vi "Move_Arm_to_Card_Pickup3.vi"(9 "index":i32=19, 10 "error in":errorcluster, 11 "Machine In":refnum<visa-resource-name>) -> (0 "X Coordinate":dbl, 1 "Y Coordinate":dbl, 2 "error out":errorcluster, 3 "Machine Out":refnum<visa-resource-name>, 4 "Z Coordinate":dbl=5.0)   [LabVIEW 2018]
doc: "Example interface for controlling uArm Swift Pro."
panel:
  in  "Write Buffer":string="G90 G0 X1\n"
  out "read buffer":string
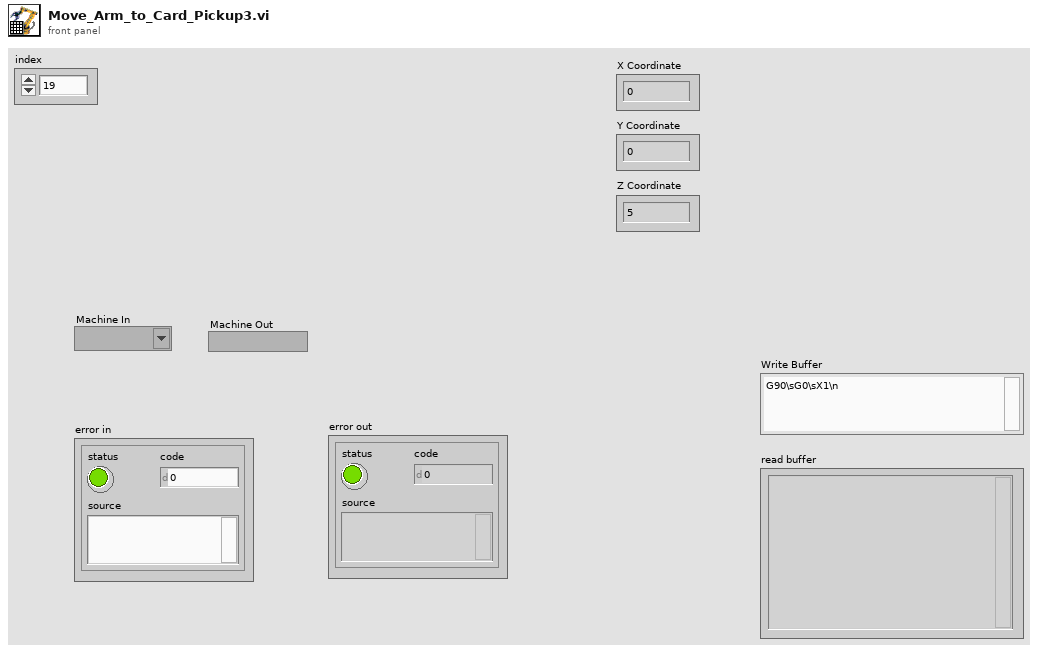
[diagram p1: front panel]
types:
  T1 = cluster{"Numeric Control":dbl, "Numeric Control":dbl}[]
  T2 = cluster{"Numeric Control":dbl, "Numeric Control":dbl}
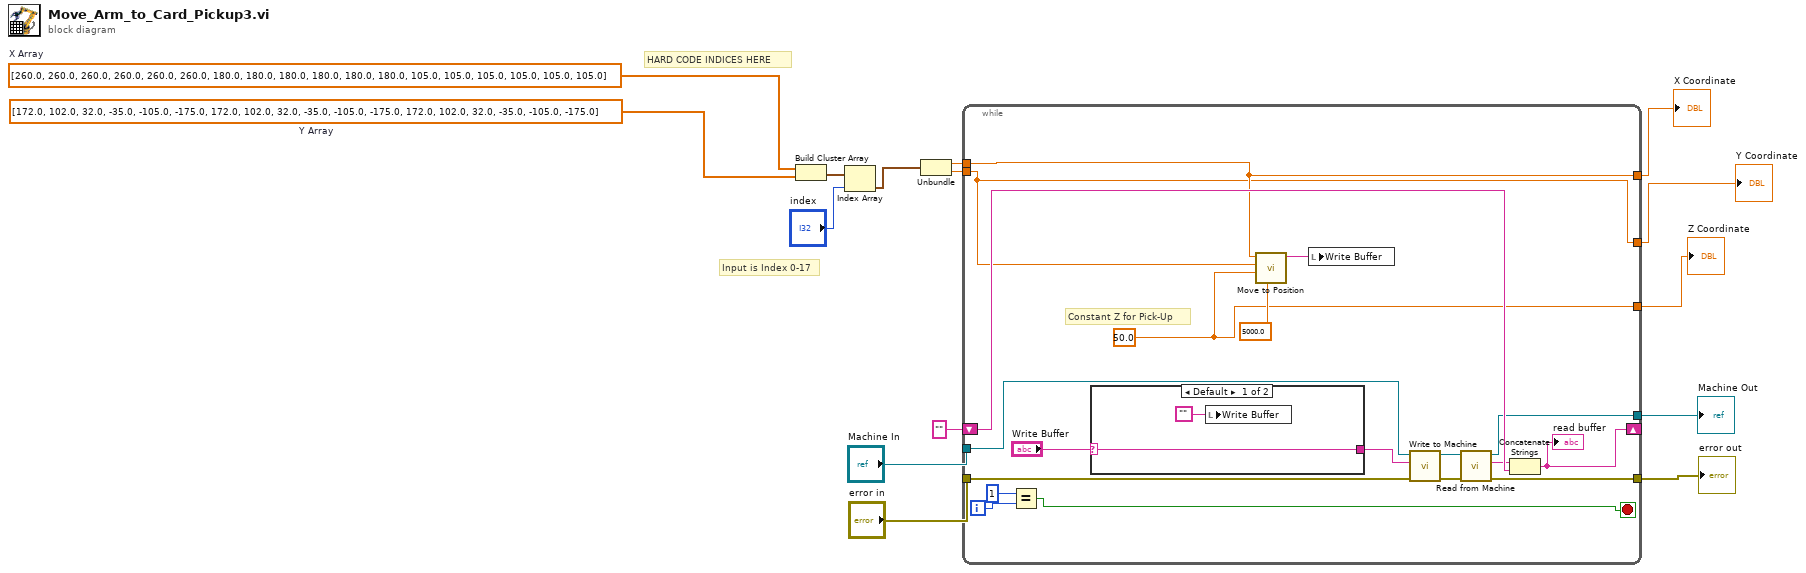
[diagram p0: block diagram]
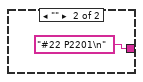
[diagram p2: hidden frame]
diagram:
  w13 = dbl[] [172.0, 102.0, 32.0, -35.0, -105.0, -175.0, 172.0, 102.0, 32.0, -35.0, -105.0, -175.0, 172.0, 102.0, 32.0, -35.0, -105.0, -175.0]  # Y Array
  w14 = dbl[] [260.0, 260.0, 260.0, 260.0, 260.0, 260.0, 180.0, 180.0, 180.0, 180.0, 180.0, 180.0, 105.0, 105.0, 105.0, 105.0, 105.0, 105.0]  # X Array
  # "HARD CODE INDICES HERE"
  # "Input is Index 0-17"
  n1 = Build Cluster Array(w14, w13) -> (w12:T1)
  n2 = Index Array(array=w12, index="index") -> (element=w11:T2)
  n3 = Unbundle(w11) -> ("Numeric Control"=w9:dbl, "Numeric Control"=w10:dbl)
  n4 = while {
    tunnel: "Machine In" -> [w32]
    tunnel: "error in" -> [w29]
    shift-right: [w30] -> _
    shift-left: "" -> [w31]
    tunnel: [w28] -> w5
    tunnel: [w24] -> w4
    tunnel: w10 -> [w16]
    tunnel: w9 -> [w17]
    tunnel: [w17] -> w3
    tunnel: [w16] -> w2
    tunnel: [w18] -> w1
    i -> [w21]
    stop <- w19 stop-if-true
    w18 = 50.0 ("Z-Position")
    # "Constant Z for Pick-Up"
    n5 = Equal?(x=1, y=w21) -> (x = y?=w19:bool)
    n6 = case shown="Default" "Write Buffer" {
      selector: "Write Buffer" -> [w36 _]
      tunnel: [w36 "#22 P2201\n"] -> w33
      frame Default {
        n7 = local write "Write Buffer"("") -> ()
      }
      frame "" {
      }
    }
    n8 = call "Move to Position.vi"("Speed"=5000.0, "Z-Position"=w18, "Y-Position"=w16, "X-Position"=w17) -> ("G-Code String"=w23:string)  [unwired: 7 in]
    n9 = local write "Write Buffer"(w23) -> ()
    n10 = call "Write to Machine .vi"("error in (no error)"=w29, "G-Code String In"=w33, "Machine In"=w32) -> ("error out"=w26:errorcluster, "Machine Out"=w25:refnum<visa-resource-name>)  [unwired: 7 in]
    n11 = call "Read from Machine.vi"("error in (no error)"=w26, "Machine In"=w25) -> ("error out"=w24:errorcluster, "read buffer"=w27:string, "Machine Out"=w28:refnum<visa-resource-name>)  [unwired: 7 in]
    n12 = Concatenate Strings(w27, w31) -> (w30:string)
    "read buffer" <- w30
  }
  "Machine Out" <- w5
  "error out" <- w4
  "Y Coordinate" <- w2
  "X Coordinate" <- w3
  "Z Coordinate" <- w1
